vi "Konfig Gasflasche aktiv.vi"(8 "error in (no error)":errorcluster caption="Fehler (Eingang, kein Fehler)", 10 "Konfig Gasflasche":bool, 11 "Referenz Gasflasche":refnum<vi>) -> (0 "error out":errorcluster caption="Fehler (Ausgang)")   [LabVIEW 2020, in "System Einstellungen V2.lvlib"]
uses:
  System Einstellungen V2.lvlib
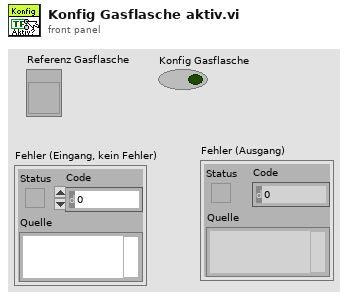
[diagram p1: front panel]
types:
  T1 = enum8{"Enabled", "Disabled", "Disabled and Grayed Out"}
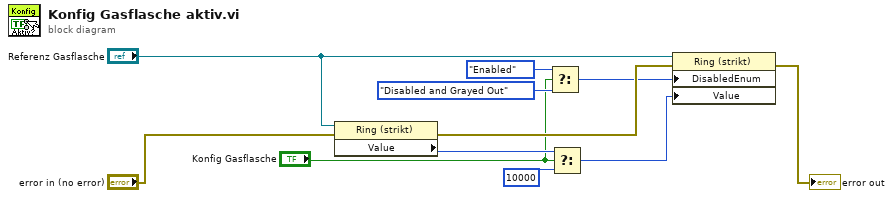
[diagram p0: block diagram]
diagram:
  n1 = property on="Eigenschaftsknoten" class="Ring (strikt)"(reference="Referenz Gasflasche", error in="error in (no error)") -> (error out=w9:errorcluster, "Value"=w10:u16)  [unwired: 1 out]
  n2 = Select(t=T1."Enabled" ("Deaktiviert"), s="Konfig Gasflasche", f=T1."Disabled and Grayed Out" ("Deaktiviert")) -> (s? t:f=w5:T1)
  n3 = Select(t=w10, s="Konfig Gasflasche", f=u16 10000) -> (s? t:f=w8:u16)
  n4 = property on="Eigenschaftsknoten" class="Ring (strikt)"(reference="Referenz Gasflasche", error in=w9, "DisabledEnum"=w5, "Value"=w8) -> (error out=→"error out":errorcluster)  [unwired: 1 out]
